vi "Abort.vi"(8 "error in (no error)":errorcluster, 11 "VISA resource name":refnum<visa-resource-name>) -> (0 "error out":errorcluster, 3 "VISA resource name out":refnum<visa-resource-name>)   [LabVIEW 2023, in "RIGOL DS1054Z Driver.lvlib"]
doc: "Aborts an acquisition.\n\n<B>Note:</B>\n Use this VI only with other low-level VIs."
uses:
  <instrlib>/RIGOL-DS1054Z-LabVIEW/RIGOL DS1054Z Driver.lvlib
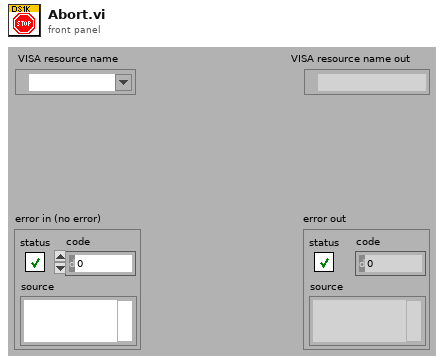
[diagram p1: front panel]
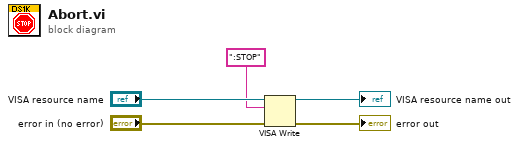
[diagram p0: block diagram]
diagram:
  n1 = VISA Write(VISA resource name="VISA resource name", write buffer=":STOP", error in (no error)="error in (no error)") -> (VISA resource name out=→"VISA resource name out":refnum<visa-resource-name>, error out=→"error out":errorcluster)  [unwired: 1 out]
